vi "Status Instrument.vi"(0 "VISA resource name":refnum<visa-resource-name>, 7 "error in (no error)":errorcluster) -> (10 "Lock-Out Code":dbl min=0.0 max=999.0 step=1.0, 11 "Beeper Status":bool, 12 "Lock-Out":bool, 13 "Beeper Enabled/Disabled":bool, 14 "Ext Scanner\nAutoscan Interval":dbl=2.0 min=2.0 max=200.0 step=1.0, 15 "Remote Interface\nMode":u16(ring) items=["Local", "Remote", "Remote w/ Lockout"], 16 "External Scanner\nInput":dbl=1.0 min=1.0 max=16.0 step=1.0, 17 "Keypad Status":bool, 18 "External Scanner\nMode (Off:0)":u16(ring) items=["Off", "Manual", "Autoscan", "Slave"], 19 "Milliseconds":dbl min=0.0 max=999.0 step=1.0, 20 "VISA resource name out":refnum<visa-resource-name>, 21 "Month":u16(ring) items=["January", "February", "March", "April", "May", "June", "Jule", "August", "September", "October", "November", "December"], 22 "Day":dbl=1.0 min=1.0 max=31.0 step=1.0, 23 "Year":dbl=1996.0 min=1996.0 max=9999.0 step=1.0, 24 "Hour":dbl min=0.0 max=23.0 step=1.0, 25 "Minutes":dbl min=0.0 max=59.0 step=1.0, 26 "Seconds":dbl min=0.0 max=59.0 step=1.0, 27 "error out":errorcluster)   [LabVIEW 2020, in "Lake Shore Cryotronics 340.lvlib"]
doc: "This VI displays various instrument settings. Parameters indicated are;\nRemote interface status\nKeypad lock-out status\nExternal scanner mode\nAudible beeper status\nKeypad status\nLogging status\nDate & Time status"
uses:
  Lake Shore Cryotronics 340.lvlib
panel:
  # "Keypad Lock-Out"
  # "Date & Time"
  # "Beeper"
  # "External Scanner"
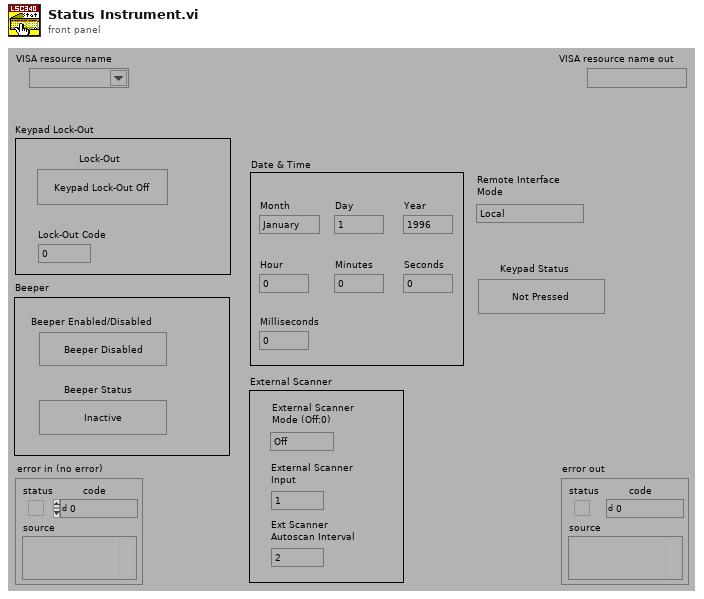
[diagram p1: front panel]
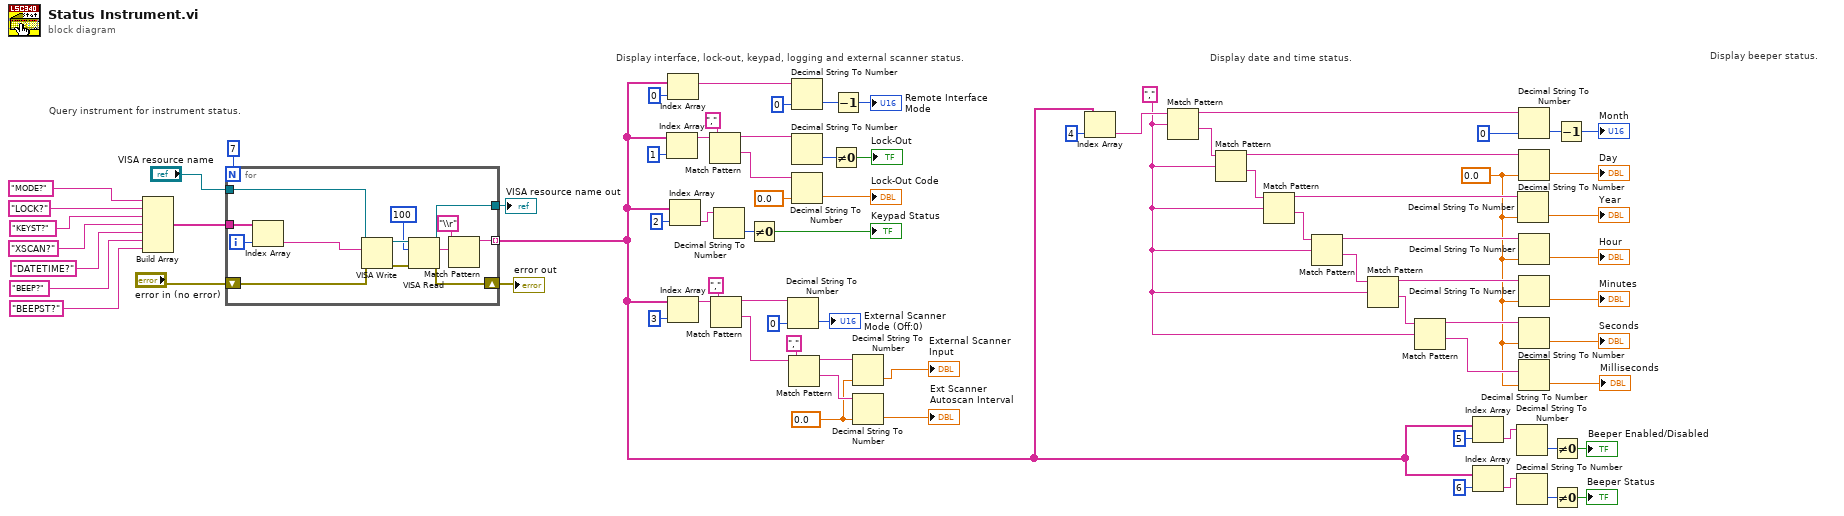
[diagram p0: block diagram]
diagram:
  w4 = 0.0 ("default (0L)")
  w5 = 0.0 ("default (0L)")
  w2 = ","
  # "Display beeper status."
  # "Display date and time status."
  # "Display interface, lock-out, keypad, logging and external scanner status."
  # "Query instrument for instrument status."
  n1 = Build Array("MODE?", "LOCK?", "KEYST?", "XSCAN?", "DATETIME?", "BEEP?", "BEEPST?") -> (w69:string[])
  n2 = for {
    N: 7 -> [_]
    tunnel: w69 -> [w80]
    shift-right: [w85] -> w77
    shift-left: "error in (no error)" -> [w86]
    tunnel: [w84] -> w78
    tunnel: "VISA resource name" -> [w83]
    tunnel: [w81] -> w8 mode=indexing
    i -> [w87]
    n3 = Index Array(array=w80, index=w87) -> (element=w79:string)
    n4 = VISA Write(VISA resource name=w83, write buffer=w79, error in (no error)=w86) -> (VISA resource name out=w91:refnum<visa-resource-name>, error out=w90:errorcluster)  [unwired: 1 out]
    n5 = VISA Read(VISA resource name=w91, byte count=100, error in (no error)=w90) -> (VISA resource name out=w84:refnum<visa-resource-name>, read buffer=w88:string, error out=w85:errorcluster)  [unwired: 1 out]
    n6 = Match Pattern(string=w88, regular expression="\\r") -> (before substring=w81:string)  [unwired: 1 in, 3 out]
  }
  "VISA resource name out" <- w78
  "error out" <- w77
  n7 = Index Array(array=w8, index=1) -> (element=w45:string)
  n8 = Index Array(array=w8, index=0) -> (element=w42:string)
  n9 = Index Array(array=w8, index=3) -> (element=w56:string)
  n10 = Index Array(array=w8, index=2) -> (element=w52:string)
  n11 = Match Pattern(string=w45, regular expression=",") -> (before substring=w46:string, after substring=w47:string)  [unwired: 1 in, 2 out]
  n12 = Match Pattern(string=w56, regular expression=",") -> (before substring=w57:string, after substring=w60:string)  [unwired: 1 in, 2 out]
  n13 = Decimal String To Number(string=w52) -> (number=w53:i32)  [unwired: 2 in, 1 out]
  n14 = Not Equal To 0?(x=w53) -> (x != 0?=→"Keypad Status":bool)
  n15 = Decimal String To Number(string=w57, default (0L)=u16 0) -> (number=→"External Scanner\nMode (Off:0)":u16)  [unwired: 1 in, 1 out]
  n16 = Match Pattern(string=w60, regular expression=",") -> (before substring=w61:string, after substring=w62:string)  [unwired: 1 in, 2 out]
  n17 = Decimal String To Number(string=w42, default (0L)=u16 0) -> (number=w41:u16)  [unwired: 1 in, 1 out]
  n18 = Decimal String To Number(string=w46) -> (number=w48:i32)  [unwired: 2 in, 1 out]
  n19 = Decimal String To Number(string=w47, default (0L)=0.0) -> (number=→"Lock-Out Code":dbl)  [unwired: 1 in, 1 out]
  n20 = Not Equal To 0?(x=w48) -> (x != 0?=→"Lock-Out":bool)
  n21 = Decrement(x=w41) -> (x-1=→"Remote Interface\nMode":u16)
  n22 = Decimal String To Number(string=w61, default (0L)=w5) -> (number=→"External Scanner\nInput":dbl)  [unwired: 1 in, 1 out]
  n23 = Decimal String To Number(string=w62, default (0L)=w5) -> (number=→"Ext Scanner\nAutoscan Interval":dbl)  [unwired: 1 in, 1 out]
  n24 = Index Array(array=w8, index=4) -> (element=w17:string)
  n25 = Match Pattern(string=w17, regular expression=w2) -> (before substring=w18:string, after substring=w25:string)  [unwired: 1 in, 2 out]
  n26 = Match Pattern(string=w25, regular expression=w2) -> (before substring=w20:string, after substring=w27:string)  [unwired: 1 in, 2 out]
  n27 = Match Pattern(string=w27, regular expression=w2) -> (before substring=w21:string, after substring=w29:string)  [unwired: 1 in, 2 out]
  n28 = Match Pattern(string=w29, regular expression=w2) -> (before substring=w22:string, after substring=w32:string)  [unwired: 1 in, 2 out]
  n29 = Match Pattern(string=w32, regular expression=w2) -> (before substring=w23:string, after substring=w34:string)  [unwired: 1 in, 2 out]
  n30 = Match Pattern(string=w34, regular expression=w2) -> (before substring=w33:string, after substring=w35:string)  [unwired: 1 in, 2 out]
  n31 = Index Array(array=w8, index=5) -> (element=w15:string)
  n32 = Index Array(array=w8, index=6) -> (element=w11:string)
  n33 = Decimal String To Number(string=w15) -> (number=w14:i32)  [unwired: 2 in, 1 out]
  n34 = Decimal String To Number(string=w11) -> (number=w13:i32)  [unwired: 2 in, 1 out]
  n35 = Decimal String To Number(string=w21, default (0L)=w4) -> (number=→"Year":dbl)  [unwired: 1 in, 1 out]
  n36 = Decimal String To Number(string=w18, default (0L)=u16 0) -> (number=w24:u16)  [unwired: 1 in, 1 out]
  n37 = Decimal String To Number(string=w20, default (0L)=w4) -> (number=→"Day":dbl)  [unwired: 1 in, 1 out]
  n38 = Decimal String To Number(string=w22, default (0L)=w4) -> (number=→"Hour":dbl)  [unwired: 1 in, 1 out]
  n39 = Decimal String To Number(string=w23, default (0L)=w4) -> (number=→"Minutes":dbl)  [unwired: 1 in, 1 out]
  n40 = Decimal String To Number(string=w33, default (0L)=w4) -> (number=→"Seconds":dbl)  [unwired: 1 in, 1 out]
  n41 = Decimal String To Number(string=w35, default (0L)=w4) -> (number=→"Milliseconds":dbl)  [unwired: 1 in, 1 out]
  n42 = Not Equal To 0?(x=w14) -> (x != 0?=→"Beeper Enabled/Disabled":bool)
  n43 = Not Equal To 0?(x=w13) -> (x != 0?=→"Beeper Status":bool)
  n44 = Decrement(x=w24) -> (x-1=→"Month":u16)
